vi "Analog DAQ_Launch.vi"(0 "DAQmx Physical Channel":tag, 9 "Timeout":i32=1000 format="%dmsec", 11 "error in":errorcluster) -> (4 "FTW Actor Connector":refnum<class "FTW-ActorConnector.lvclass">, 6 "Initialized Response":string, 8 "Instance Inbox Address":string, 15 "error out":errorcluster)   [LabVIEW 2018]
uses:
  source/actor/Connector/FTW-ActorConnector.lvclass
  Core/Analog DAQ-Core_Process.vi
  Core/Analog DAQ-Core.lvclass
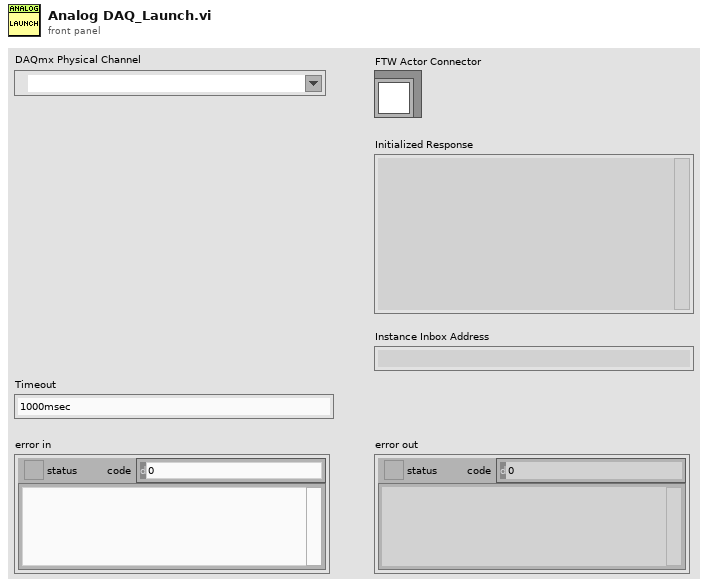
[diagram p1: front panel]
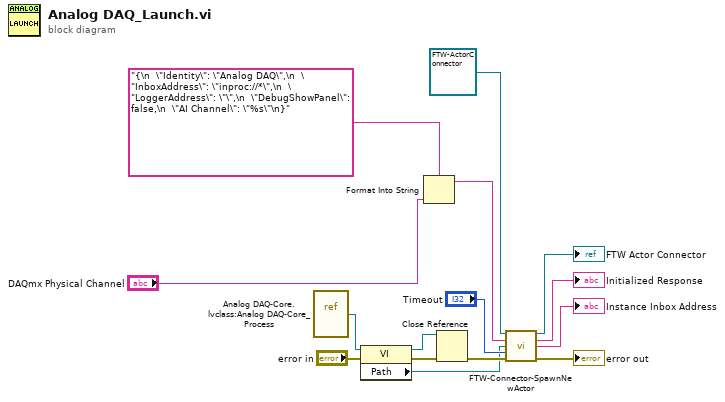
[diagram p0: block diagram]
diagram:
  n1 = vi-ref "Analog DAQ-Core.lvclass:Analog DAQ-Core_Process.vi"() -> (w9:refnum<vi>)
  n2 = property class="VI"(reference=w9, error in="error in") -> (reference out=w8:refnum<vi>, error out=w7:errorcluster, "Path"=w4:path)
  n3 = Format Into String(format string="{\n  \"Identity\": \"Analog DAQ\",\n  \"InboxAddress\": \"inproc://*\",\n  \"LoggerAddress\": \"\",\n  \"DebugShowPanel\": false,\n  \"AI Channel\": \"%s\"\n}" ("Configuration"), "DAQmx Physical Channel") -> (resulting string=w2:string)  [unwired: 2 in, 1 out]
  n4 = Close Reference(reference=w8, error in (no error)=w7) -> (error out=w5:errorcluster)
  n5 = call "FTW-Connector-SpawnNewActor.vi"("FTW Actor Connector Type"=refnum<class "FTW-ActorConnector.lvclass"> refnum ("TTK_Splashscreen.lvclass"), "Configuration"=w2, "Actor VI Filepath"=w4, "Timeout"="Timeout", "error in"=w5) -> ("FTW Actor Connector"=→"FTW Actor Connector":refnum<class "FTW-ActorConnector.lvclass">, "Initialized Response"=→"Initialized Response":string, "Instance Inbox Address"=→"Instance Inbox Address":string, "error out"=→"error out":errorcluster)  [unwired: 7 in]
